vi "Protection_Valid_Calculation.vi"(7 "Value Received":dbl, 8 "error in":errorcluster, 9 "Signal Valid Values In":dbl[](array[numeric]), 10 "Signal Settings":T1 {"Protection Configuration"."CRC Channels"."Data Type" items=["Signed", "Unsigned", "IEEE Float"]}, 11 "Signal Values In":dbl[](array[numeric])) -> (0 "error out":errorcluster, 1 "Signal Valid Values Out":dbl[](array[numeric]), 3 "Signal Values Out":dbl[](array[numeric]))   [LabVIEW 2019]
uses:
  <vilib>/xnet/xnet.llb/XNET Convert (Signal to Frame Raw).vi
  <vilib>/NI VeriStand/Custom Device Tools/Custom Device Utility Library/Custom Device Utility Library.lvlib
  SubModules/Frame-Protection-Support/Source/Shared/Types/Exported Counter Settings.ctl
  SubModules/Frame-Protection-Support/Source/Shared/Protection and Counter Support Shared.lvlib
  SubModules/Frame-Protection-Support/Source/Shared/Types/XNET Signal Configuration.ctl
  SubModules/Frame-Protection-Support/Source/Shared/Types/Protection Type.ctl
  SubModules/Frame-Protection-Support/Source/Engine/Types/RT Protection Configuration.ctl
  SubModules/Frame-Protection-Support/Source/Engine/Protection and Counter Support Engine.lvlib
  SubModules/Frame-Protection-Support/Source/Shared/Types/RT Exported Signal Settings.ctl
panel:
  out "Value Calculated":u8
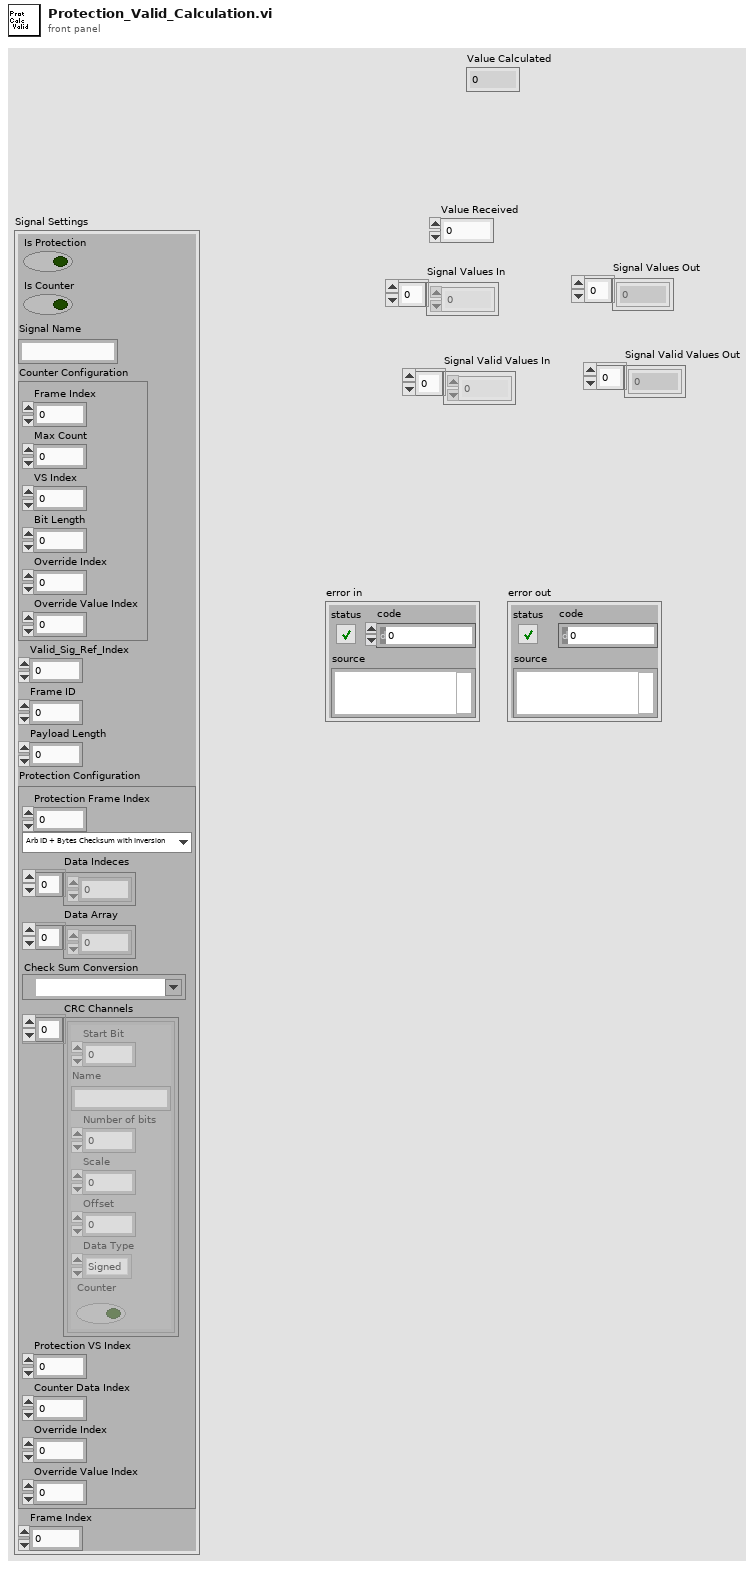
[diagram p1: front panel]
types:
  T1 = typedef "RT Exported Signal Settings.ctl" = cluster{"Is Protection":bool, "Is Counter":bool, "Signal Name":string, "Counter Configuration":T2, "Valid_Sig_Ref_Index":i32, "Frame ID":u32, "Payload Length":u32, "Protection Configuration":T3, "Frame Index":i32}
  T2 = typedef "Protection and Counter Support Shared.lvlib/Exported Counter Settings.ctl" = cluster{"Frame Index":i32, "Max Count":dbl, "VS Index":i32, "Bit Length":i64, "Override Index":i32, "Override Value Index":i32}
  T3 = typedef "Protection and Counter Support Engine.lvlib/RT Protection Configuration.ctl" = cluster{"Protection Frame Index":i32, "Protection Type":T4, "Data Indeces":i32[], "Data Array":dbl[], "Check Sum Conversion":refnum<k21>, "CRC Channels":T5[], "Protection VS Index":i32, "Counter Data Index":i32, "Override Index":i32, "Override Value Index":i32}
  T4 = typedef "Protection and Counter Support Shared.lvlib/Protection Type.ctl" = enum16{"Arb ID + Bytes Checksum with Inversion", "Arb ID + Bytes CRC with Inversion", "Reversed Raw Signal Checksum with Inversion", "Concatenated Two's Compliment"}
  T5 = typedef "Protection and Counter Support Shared.lvlib/XNET Signal Configuration.ctl" = cluster{"Start Bit":i32, "Name":string, "Number of bits":i32, "Scale":dbl, "Offset":dbl, "Data Type":u32, "Counter":bool}
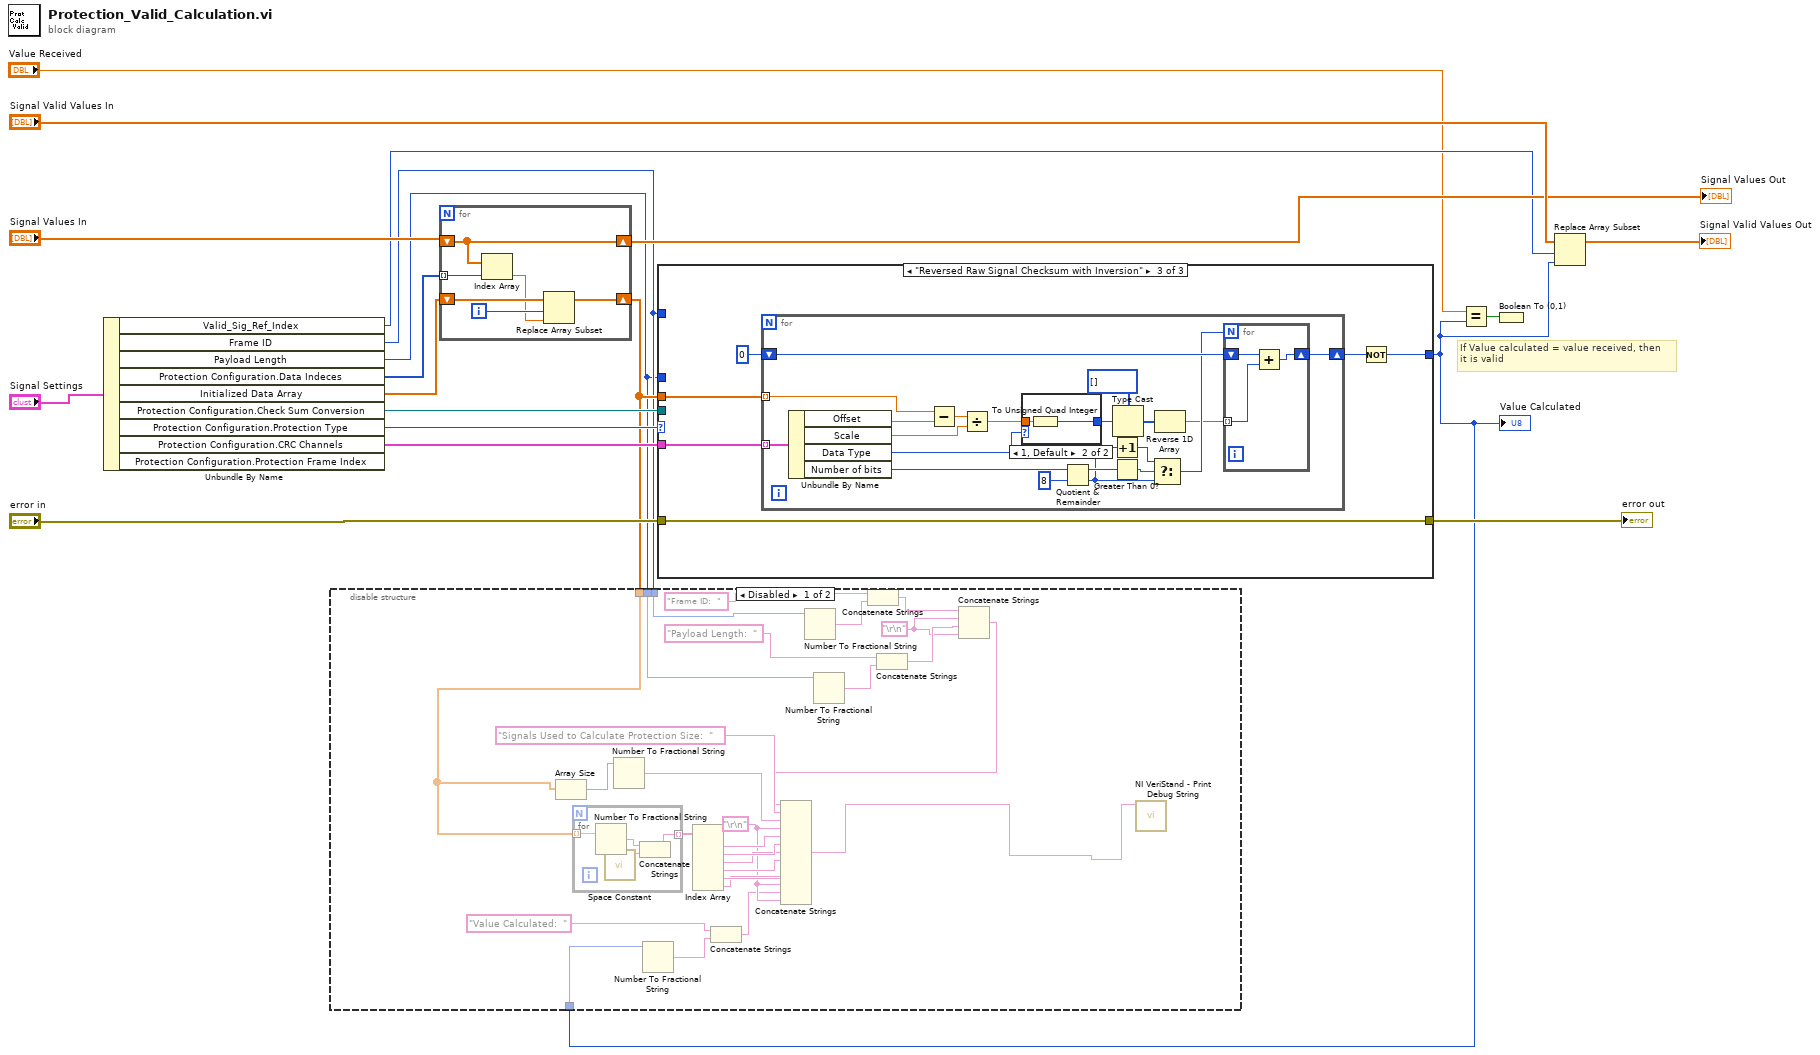
[diagram p0: block diagram]
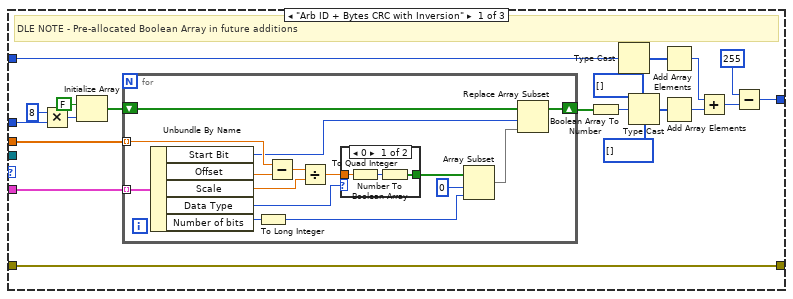
[diagram p3: hidden frame]
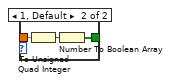
[diagram p4: hidden frame]
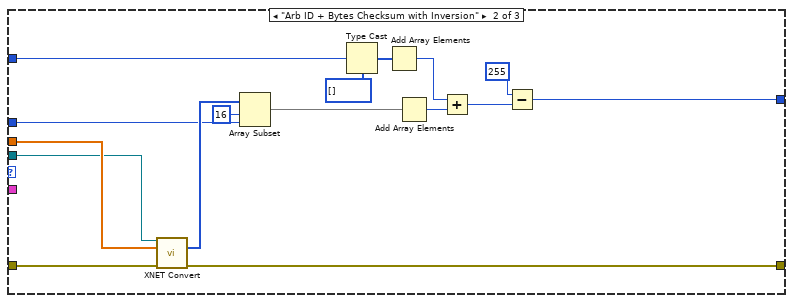
[diagram p5: hidden frame]
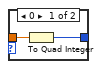
[diagram p6: hidden frame]
diagram:
  # "If Value calculated = value received, then\nit is valid"
  n1 = Unbundle By Name("Signal Settings") -> ("Valid_Sig_Ref_Index"=w6:i32, "Frame ID"=w2:u32, "Payload Length"=w1:u32, "Protection Configuration.Data Indeces"=w15:i32[], "Initialized Data Array"=w14:dbl[], "Protection Configuration.Check Sum Conversion"=w12:refnum<k21>, "Protection Configuration.Protection Type"=w13:T4, "Protection Configuration.CRC Channels"=w16:T5[])  [unwired: 1 out]
  n2 = for {
    shift-right: [w24] -> w8
    shift-left: "Signal Values In" -> [w24]
    tunnel: w15 -> [w25] mode=indexing
    shift-right: [w20] -> w4
    shift-left: w14 -> [w23]
    i -> [w22]
    n3 = Index Array(array=w24, index=w25) -> (element=w21:dbl)
    n4 = Replace Array Subset(array=w23, new element=w21, index=w22) -> (w20:dbl[])
  }
  "Signal Values Out" <- w8
  n5 = case shown="\"Reversed Raw Signal Checksum with Inversion\"" w13 {
    tunnel: w2 -> [w43 w68 _]
    tunnel: [w38 w76 w84] -> w3
    tunnel: "error in" -> [w34 w75 w83]
    tunnel: [w34 w70 w83] -> w18
    tunnel: w16 -> [w32 _ w86]
    tunnel: w4 -> [w33 w73 w85]
    tunnel: w12 -> [_ w72 _]
    tunnel: w1 -> [w28 w67 _]
    frame "Arb ID + Bytes CRC with Inversion" {
      # "DLE NOTE - Pre-allocated Boolean Array in future additions"
      n6 = Multiply(x=u32 8, y=w28) -> (x*y=w29:u32)
      n7 = Initialize Array(FALSE, w29) -> (w31:bool[])
      n8 = for {
        tunnel: w32 -> [w60] mode=indexing
        shift-right: [w51] -> w37
        shift-left: w31 -> [w53]
        tunnel: w33 -> [w50] mode=indexing
        n9 = Unbundle By Name(w60) -> ("Start Bit"=w47:i32, "Offset"=w59:dbl, "Scale"=w57:dbl, "Data Type"=w49:u32, "Number of bits"=w55:i32)
        n10 = To Long Integer(number=w55) -> (32bit integer=w46:i32)
        n11 = Subtract(x=w50, y=w59) -> (x-y=w58:dbl)
        n12 = Divide(x=w58, y=w57) -> (x/y=w56:dbl)
        n13 = case shown="0" w49 {
          tunnel: w56 -> [w63 w66]
          tunnel: [w61 w64] -> w48
          frame 0 {
            n14 = To Quad Integer(1:w63) -> (0:w62:i64)
            n15 = Number To Boolean Array(number=w62) -> (Boolean array=w61:bool[])
          }
          frame 1, Default {
            n16 = To Unsigned Quad Integer(1:w66) -> (0:w65:u64)
            n17 = Number To Boolean Array(number=w65) -> (Boolean array=w64:bool[])
          }
        }
        n18 = Array Subset(array=w48, index=0, length=w46) -> (w52:bool[])
        n19 = Replace Array Subset(array=w53, new element=w52, index=w47) -> (w51:bool[])
      }
      n20 = Boolean Array To Number(Boolean array=w37) -> (number=w36:u64)
      n21 = Type Cast(type=u8[] [], x=w43) -> (*(type *) &x=w42:u8[])
      n22 = Type Cast(type=u8[] [], x=w36) -> (*(type *) &x=w26:u8[])
      n23 = Add Array Elements(numeric array=w42) -> (sum=w41:u8)
      n24 = Add Array Elements(numeric array=w26) -> (sum=w45:u8)
      n25 = Add(x=w41, y=w45) -> (x+y=w40:u8)
      n26 = Subtract(x=u8 255, y=w40) -> (x-y=w38:u8)
    }
    frame "Arb ID + Bytes Checksum with Inversion" {
      n27 = call-poly <vilib>:"XNET Convert.vi"("session in"=w72, "signal data"=w73, "error in (no error)"=w75) -> ("frame data"=w69:u8[], "error out"=w70:errorcluster)  [unwired: 10 in, 1 out]
      n28 = Array Subset(array=w69, index=16 ("length"), length=w67) -> (w71:u8[])
      n29 = Type Cast(type=u8[] [], x=w68) -> (*(type *) &x=w80:u8[])
      n30 = Add Array Elements(numeric array=w80) -> (sum=w79:u8)
      n31 = Add Array Elements(numeric array=w71) -> (sum=w82:u8)
      n32 = Add(x=w79, y=w82) -> (x+y=w78:u8)
      n33 = Subtract(x=u8 255, y=w78) -> (x-y=w76:u8)
    }
    frame "Reversed Raw Signal Checksum with Inversion" {
      n34 = for {
        tunnel: w86 -> [w108] mode=indexing
        tunnel: w85 -> [w105] mode=indexing
        shift-right: [w102] -> w87
        shift-left: u8 0 -> [w103]
        n35 = Unbundle By Name(w108) -> ("Offset"=w107:dbl, "Scale"=w106:dbl, "Data Type"=w104:u32, "Number of bits"=w100:i32)
        n36 = Subtract(x=w105, y=w107) -> (x-y=w99:dbl)
        n37 = Divide(x=w99, y=w106) -> (x/y=w98:dbl)
        n38 = case shown="1, Default" w104 {
          tunnel: w98 -> [w113 w115]
          tunnel: [w112 w114] -> w101
          frame 0 {
            n39 = To Quad Integer(1:w113) -> (0:w112:i64)
          }
          frame 1, Default {
            n40 = To Unsigned Quad Integer(1:w115) -> (0:w114:u64)
          }
        }
        n41 = Quotient & Remainder(x=w100, y=8) -> (x-y*floor(x/y)=w95:i32, floor(x/y)=w93:i32)
        n42 = Increment(x=w93) -> (x+1=w94:i32)
        n43 = Greater Than 0?(x=w95) -> (x > 0?=w96:bool)
        n44 = Type Cast(type=u8[] [], x=w101) -> (*(type *) &x=w90:u8[])
        n45 = Select(t=w94, s=w96, f=w93) -> (s? t:f=w92:i32)
        n46 = Reverse 1D Array(array=w90) -> (reversed array=w89:u8[])
        n47 = for {
          N: w92 -> [_]
          tunnel: w89 -> [w110] mode=indexing
          shift-right: [w109] -> w102
          shift-left: w103 -> [w111]
          n48 = Add(x=w111, y=w110) -> (x+y=w109:u8)
        }
      }
      n49 = Not(x=w87) -> (.not. x?=w84:u8)
    }
  }
  "error out" <- w18
  "Value Calculated" <- w3
  n50 = disable-structure shown="Disabled" {
    disable-tunnel: w4 -> [w142 _]
    disable-tunnel: w3 -> [w141 _]
    disable-tunnel: w2 -> [w140 _]
    disable-tunnel: w1 -> [w139 _]
    frame Disabled {
      w117 = "\r\n"
      w127 = "\r\n"
      n51 = Array Size(array=w142) -> (size(s)=w138:i32)
      n52 = for {
        tunnel: w142 -> [w144] mode=indexing
        tunnel: [w143] -> w135 mode=indexing
        n53 = Number To Fractional String(number=w144) -> (F-format string=w146:string)  [unwired: 3 in]
        n54 = call <vilib>:"Space Constant.vi"() -> ("String"=w145:string)
        n55 = Concatenate Strings(w146, w145) -> (w143:string)
      }
      n56 = Number To Fractional String(number=w138) -> (F-format string=w136:string)  [unwired: 3 in]
      n57 = Number To Fractional String(number=w141) -> (F-format string=w125:string)  [unwired: 3 in]
      n58 = Index Array(array=w135) -> (element #1=w134:string, element #2=w133:string, element #3=w132:string, element #4=w131:string, element #5=w130:string, element #6=w129:string)  [unwired: 6 in]
      n59 = Concatenate Strings("Value Calculated:  ", w125) -> (w124:string)
      n60 = Number To Fractional String(number=w140) -> (F-format string=w122:string)  [unwired: 3 in]
      n61 = Number To Fractional String(number=w139) -> (F-format string=w121:string)  [unwired: 3 in]
      n62 = Concatenate Strings("Frame ID:  ", w122) -> (w119:string)
      n63 = Concatenate Strings("Payload Length:  ", w121) -> (w118:string)
      n64 = Concatenate Strings(w119, w117, w118, w117) -> (w116:string)
      n65 = Concatenate Strings(w116, "Signals Used to Calculate Protection Size:  ", w136, w127, w134, w133, w132, w131, w130, w129, w127, w124, w127) -> (w128:string)
      n66 = call <vilib>:"NI VeriStand - Print Debug String.vi"("Message"=w128) -> ()  [unwired: 10 in, 1 out]
    }
    frame Enabled {
    }
  }
  n67 = Equal?(x="Value Received", y=w3) -> (x = y?=w7:bool)
  n68 = Boolean To (0,1)(Boolean=w7) -> ()  [unwired: 1 out]
  n69 = Replace Array Subset(array="Signal Valid Values In", new element=w3, index=w6) -> (→"Signal Valid Values Out":dbl[])
